vi "Display name.vi"(1 "State In":T1) -> (0 "Name":string)   [LabVIEW 2018, in "IsA.xnode"]
uses:
  IsA.xnode
  State.ctl
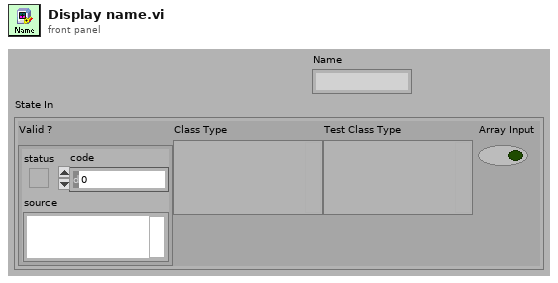
[diagram p1: front panel]
types:
  T1 = typedef "IsA.xnode/State.ctl" = cluster{"Valid ?":errorcluster, "Class Type":variant, "Test Class Type":variant, "Array Input":bool}
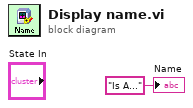
[diagram p0: block diagram]
diagram:
  "Name" <- "Is A..." ("Name")
